vi "EditUser-Window.vi"(8 "error in":errorcluster, 9 "权  限":T1, 10 "密  码":string, 11 "用户名":string) -> (0 "error out":errorcluster)   [LabVIEW 2017, in "Login-UI.lvlib"]
uses:
  Login-UI.lvlib
  User-Role.ctl
  User-Info.ctl
panel:
  in  "Exit":bool
  in  "Save":bool
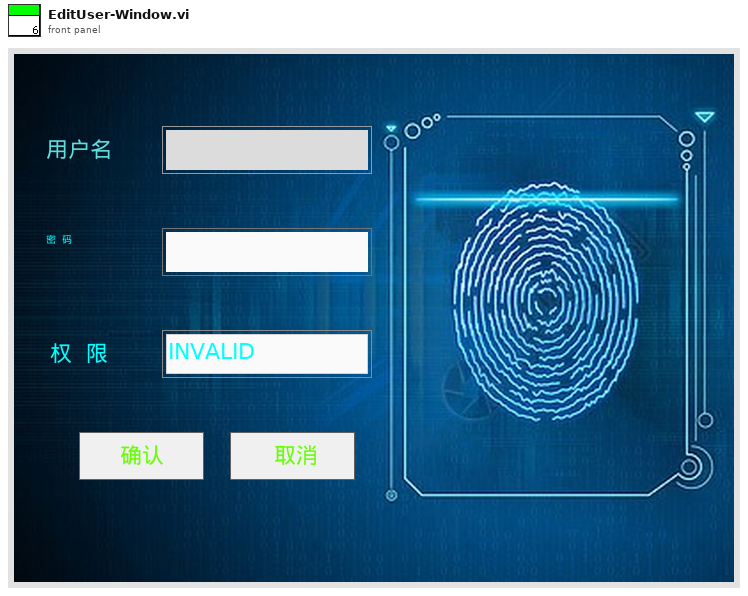
[diagram p1: front panel]
types:
  T1 = typedef "Login-UI.lvlib/User-Role.ctl" = enum16{"INVALID", "Operator", "Engineer", "Admin"}
  T2 = enum32{"Invalid", "Standard", "Closed", "Hidden", "Minimized", "Maximized"}
  T3 = enum32{"invalid app kind", "Development System", "Run Time System", "Student Edition", "Embedded LabVIEW", "Evaluation", "Custom"}
  T4 = typedef "Login-UI.lvlib/User-Info.ctl" = cluster{"UserName":string, "Password":string, "Role":T1}
  T5 = cluster{"Core":cluster{"Current VI Reference":refnum<vi>, "Close Panel on Exit?":bool}, "Your Boolean data":bool, "Your string data":string, "Cluster":T4}
  T6 = cluster{"Current VI Reference":refnum<vi>, "Close Panel on Exit?":bool}
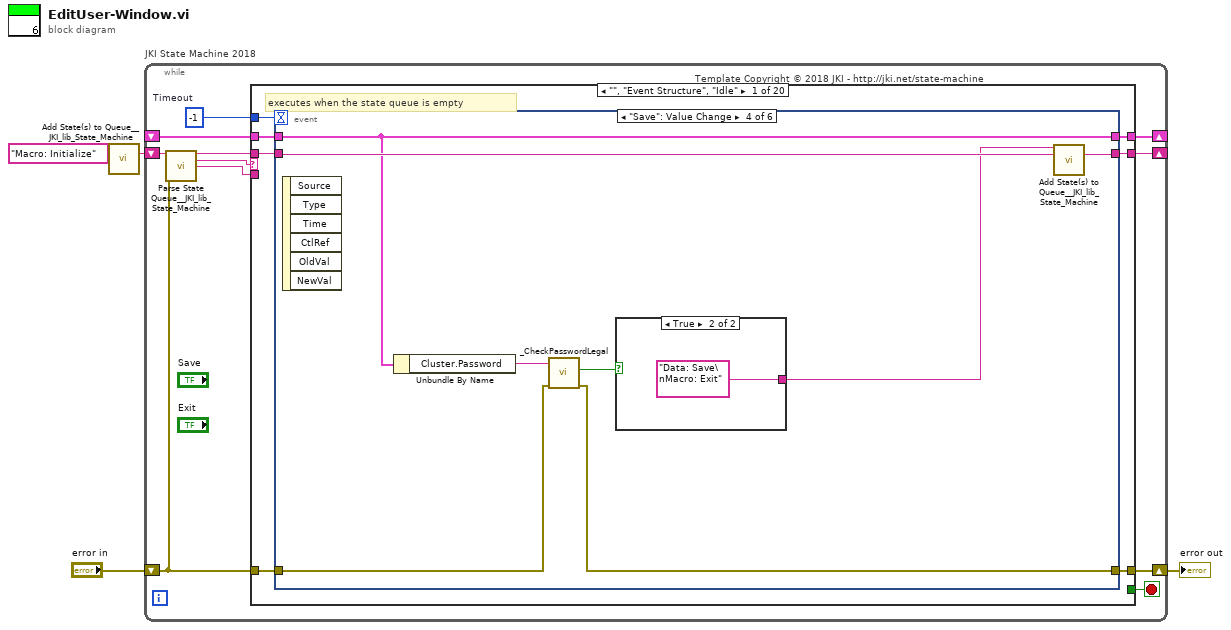
[diagram p0: block diagram]
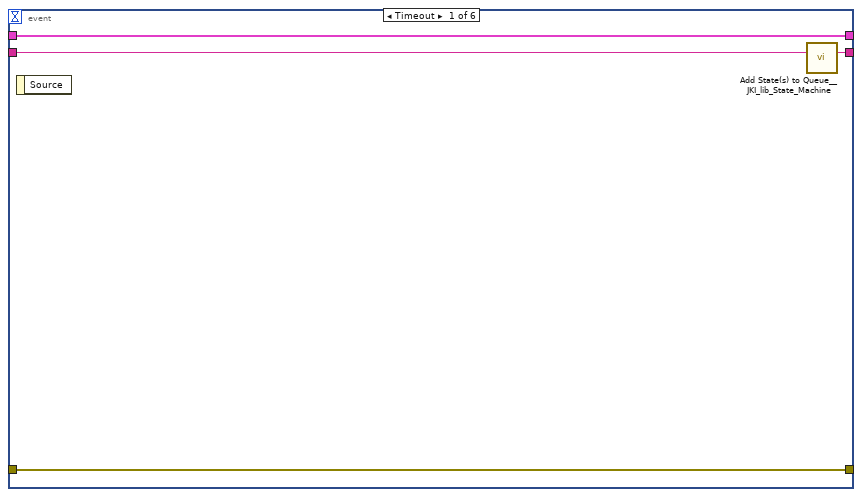
[diagram p2: hidden frame]
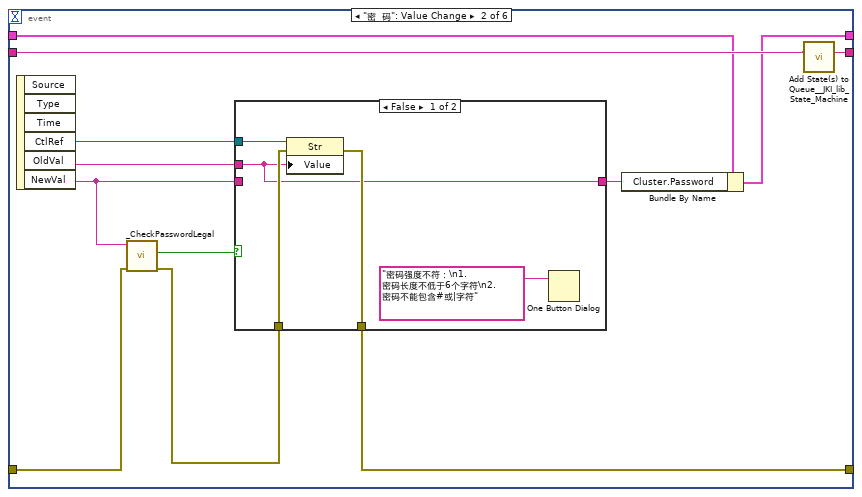
[diagram p3: hidden frame]
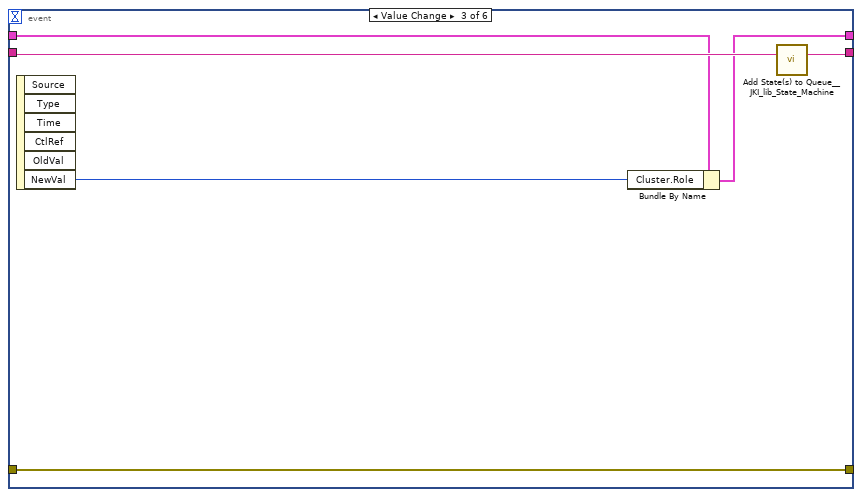
[diagram p5: hidden frame]
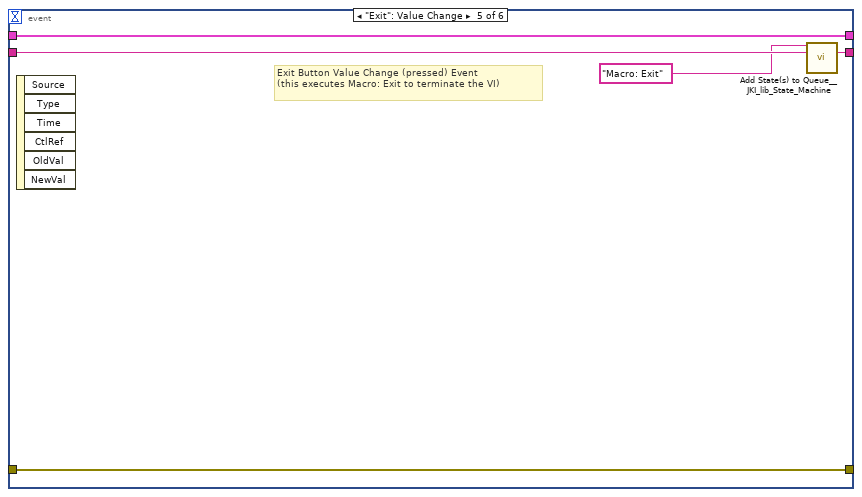
[diagram p7: hidden frame]
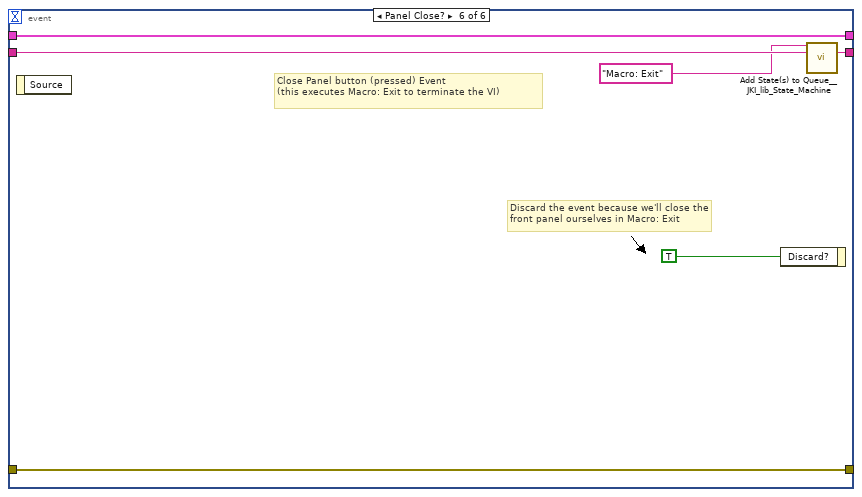
[diagram p8: hidden frame]
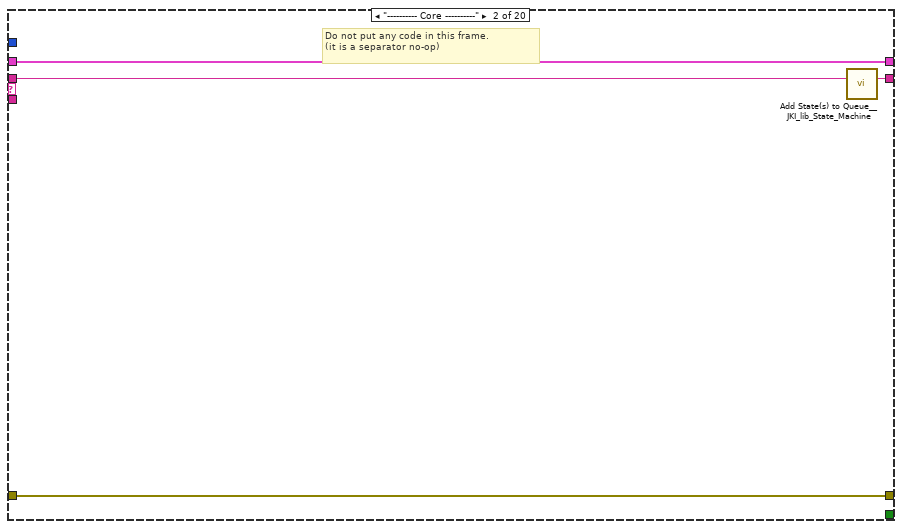
[diagram p9: hidden frame]
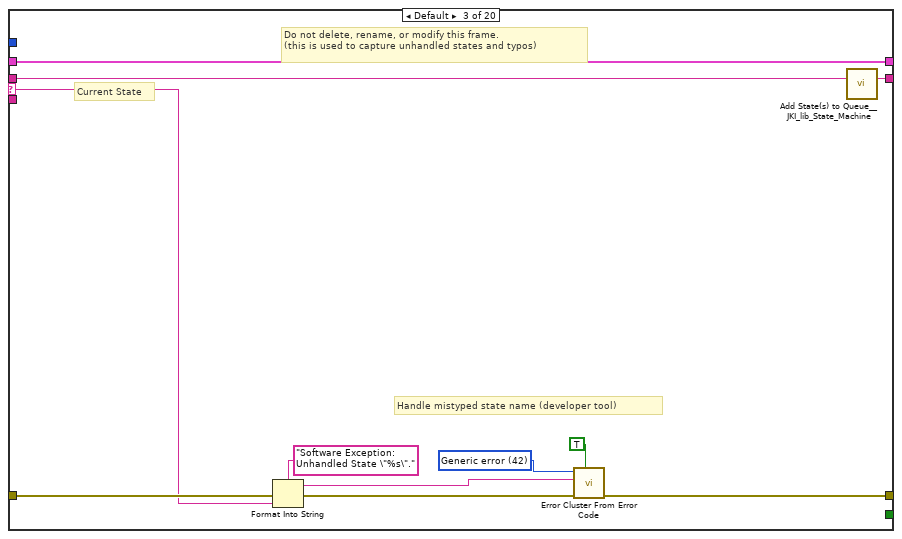
[diagram p10: hidden frame]
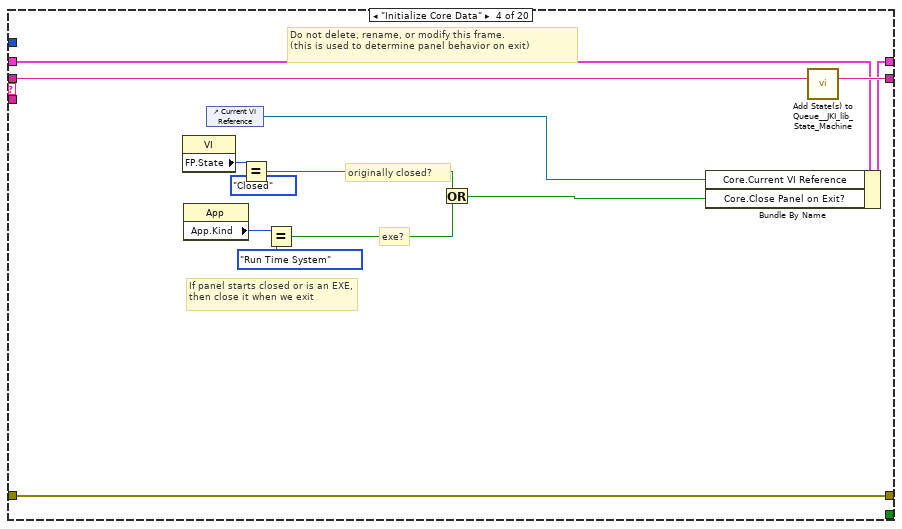
[diagram p11: hidden frame]
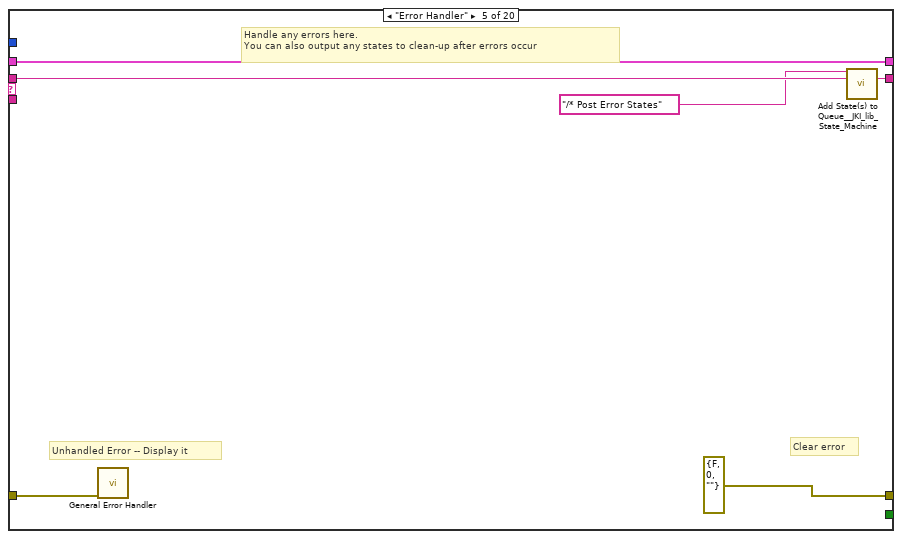
[diagram p12: hidden frame]
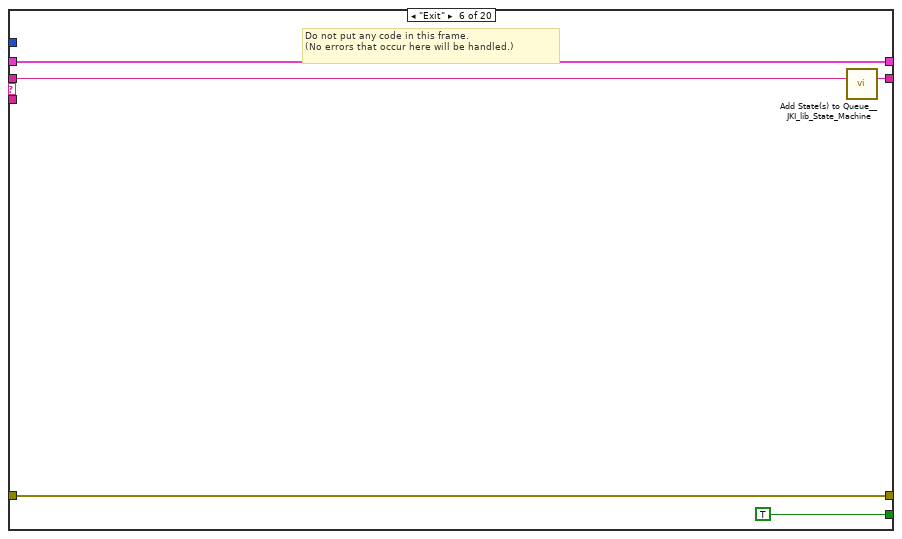
[diagram p13: hidden frame]
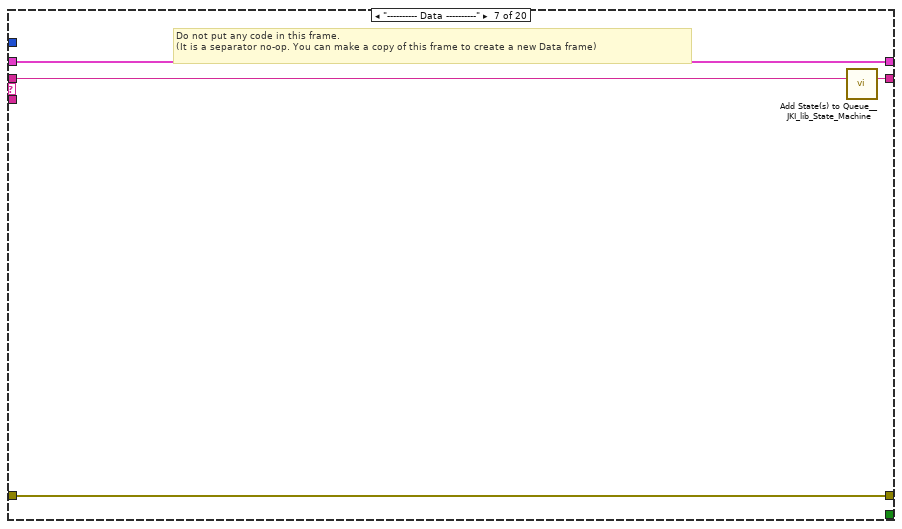
[diagram p14: hidden frame]
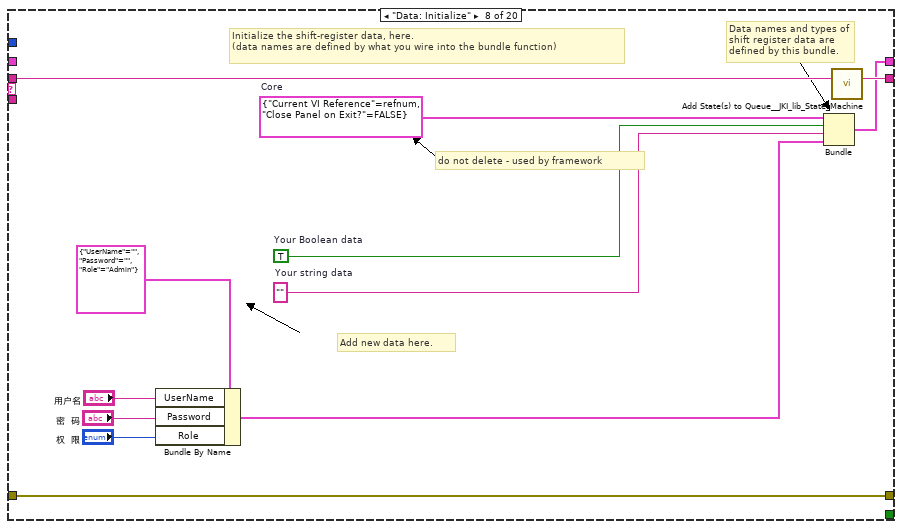
[diagram p15: hidden frame]
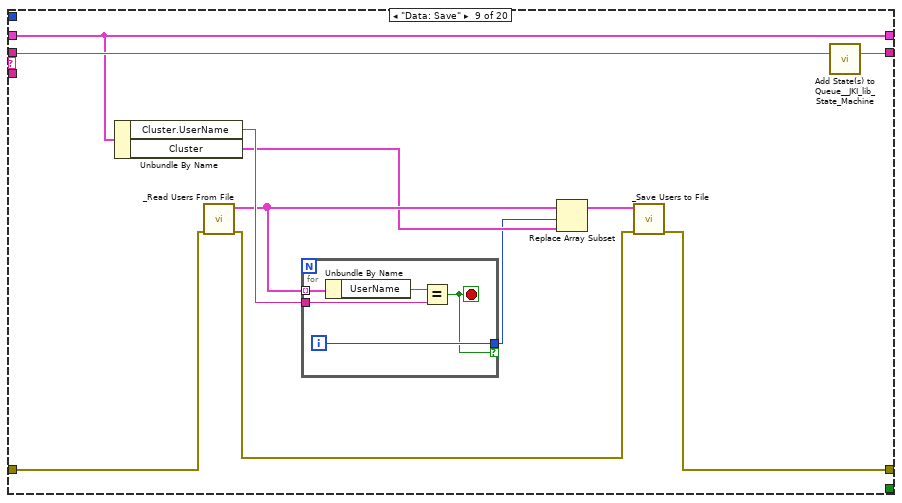
[diagram p16: hidden frame]
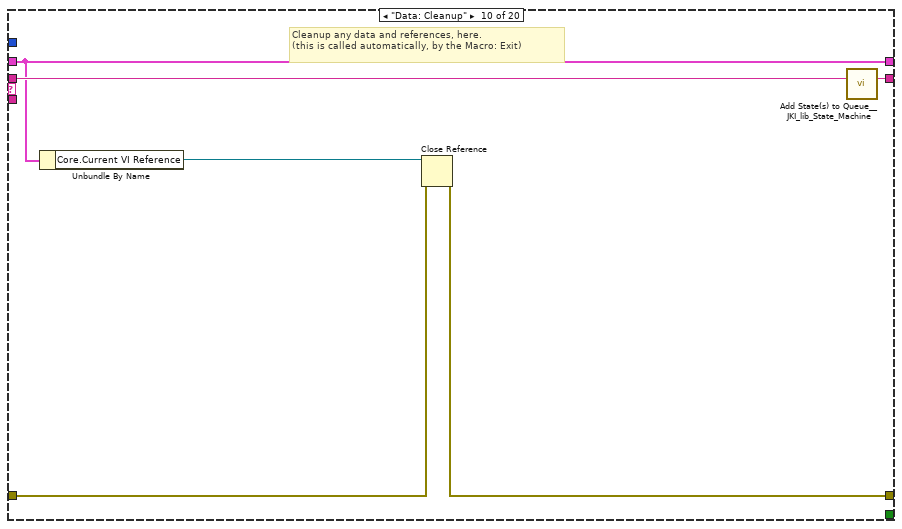
[diagram p17: hidden frame]
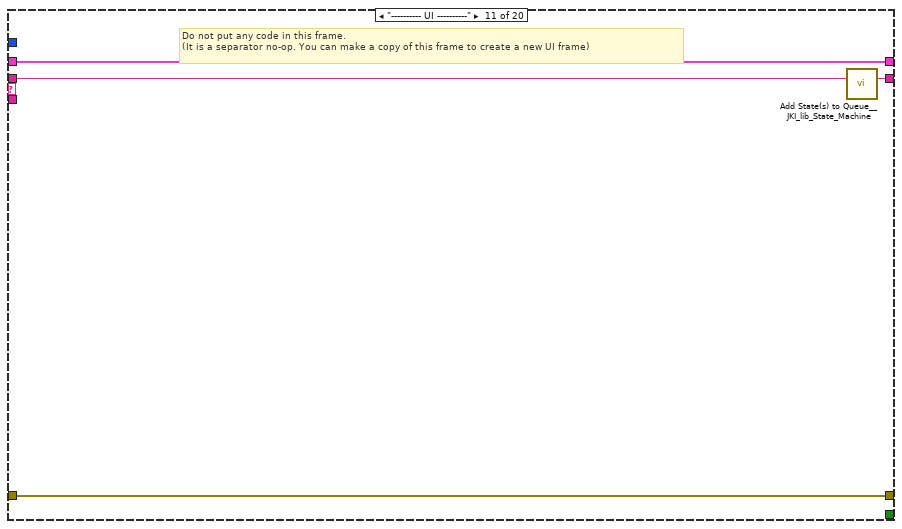
[diagram p18: hidden frame]
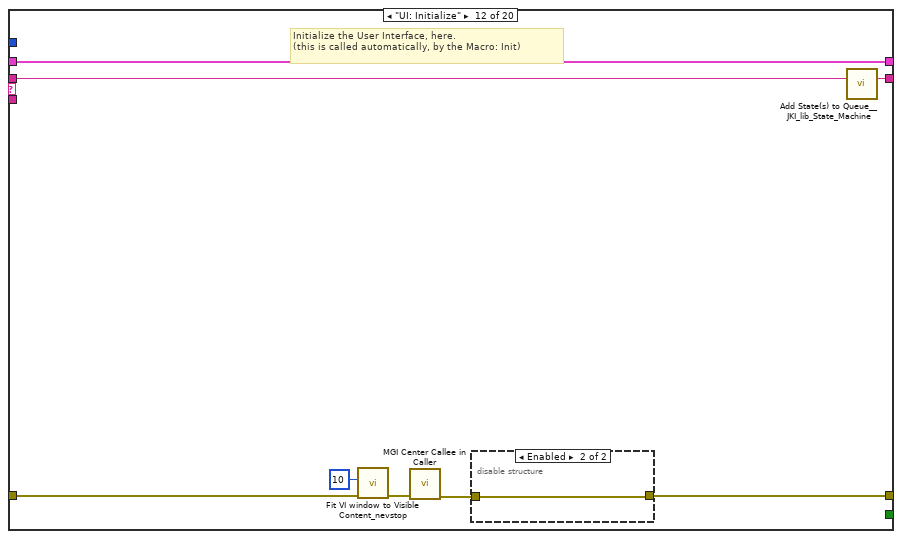
[diagram p19: hidden frame]
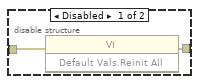
[diagram p20: hidden frame]
diagram:
  n1 = call <vilib>:"Add State(s) to Queue__JKI_lib_State_Machine.vi"("State(s) in (\"\")"="Macro: Initialize") -> ("States Out"=w4:string)  [unwired: 14 in]
  n2 = while "JKI State Machine 2018" {
    shift-right: [w8] -> _
    shift-left: _ -> [w7]
    shift-right: [w11] -> w1
    shift-left: "error in" -> [w5]
    shift-right: [w10] -> _
    shift-left: w4 -> [w12]
    stop <- w9 stop-if-true
    w6 = -1  # Timeout
    # "Template Copyright © 2018 JKI - http://jki.net/state-machine"
    n3 = call <vilib>:"Parse State Queue__JKI_lib_State_Machine.vi"("State Queue"=w12, "Error In (no error)"=w5) -> ("Remaining States"=w14:string, "Current State"=w15:string, "Arguments"=w13:string)  [unwired: 11 in]
    n4 = case shown="\"\", \"Event Structure\", \"Idle\"" w15 {
      selector: w15 -> [_ _ w76 _ _ _ _ _ _ _ _ _ _ _ _ _ _ _ _ _]
      tunnel: w14 -> [w22 w75 w80 w99 w105 w110 w114 w126 w136 w148 w152 w160 w169 w180 w249 w254 w264 w268 w272 w276]
      tunnel: w13 -> [_ _ _ _ _ _ _ _ _ _ _ _ w164 w174 _ _ _ _ _ _]
      tunnel: w7 -> [w21 w72 w78 w92 w102 w108 w111 _ w135 w143 w149 w158 w167 w176 w246 w251 w261 w265 w269 w273]
      tunnel: [w20 w73 w82 w96 errorcluster {"status"=FALSE, "code"=0, "source"=""} ("error out") w107 w112 w123 w133 w144 w150 w153 w165 w177 w247 w252 w262 w266 w270 w274] -> w11
      tunnel: w5 -> [w19 w73 w81 w96 w101 w107 w112 w123 w134 w145 w150 w155 w166 w178 w247 w252 w262 w266 w270 w274]
      tunnel: [w16 w74 w79 w98 w104 w109 w113 w125 w137 w147 w151 w159 w168 w179 w248 w253 w263 w267 w271 w275] -> w10
      tunnel: [_ _ _ _ _ TRUE _ _ _ _ _ _ _ _ _ _ _ _ _ _] -> w9
      tunnel: [w18 w72 w78 w97 w102 w108 w111 w124 w135 w143 w149 w158 w167 w176 w246 w251 w261 w265 w269 w273] -> w8
      tunnel: w6 -> [w17 _ _ _ _ _ _ _ _ _ _ _ _ _ _ _ _ _ _ _]
      frame "", "Event Structure", "Idle" {
        # "executes when the state queue is empty"
        n5 = event shown="[3] \"Save\": Value Change" {
          selector: _ -> [_ _ _ _ _ _]
          dyn-events: _ -> [_ _ _ _ _ _]
          timeout: w17 -> [_ _ _ _ _ _]
          tunnel: w22 -> [w26 w34 w49 w58 w65 w71]
          tunnel: [w25 w35 w50 w59 w64 w70] -> w16
          tunnel: w21 -> [w23 w29 w48 w56 w62 w68]
          tunnel: [w24 w36 w51 w52 w63 w69] -> w20
          tunnel: w19 -> [w24 w32 w51 w53 w63 w69]
          tunnel: [w23 w27 w47 w56 w62 w68] -> w18
          event Timeout {
            n6 = event-data() -> ()  [unwired: 1 in, 1 out]
            n7 = call <vilib>:"Add State(s) to Queue__JKI_lib_State_Machine.vi"("State(s) in (\"\")"=w26) -> ("States Out"=w25:string)  [unwired: 14 in]
          }
          event "密  码": Value Change {
            n8 = event-data() -> ("CtlRef"=w37:refnum<vi>, "OldVal"=w38:string, "NewVal"=w33:string)  [unwired: 1 in, 3 out]
            n9 = call "_CheckPasswordLegal.vi"("error in (no error)"=w32, "Password"=w33) -> ("error out"=w31:errorcluster, "legal?"=w30:bool)  [unwired: 8 in]
            n10 = case shown="False" w30 {
              tunnel: w38 -> [w39 _]
              tunnel: w33 -> [_ w44]
              tunnel: [w42 w45] -> w36
              tunnel: w37 -> [w41 _]
              tunnel: w31 -> [w40 w45]
              tunnel: [w39 w44] -> w28
              frame False {
                n11 = property class="Str"(reference=w41, error in=w40, "Value"=w39) -> (error out=w42:errorcluster)  [unwired: 1 out]
                n12 = One Button Dialog(message="密码强度不符：\n1.密码长度不低于6个字符\n2. 密码不能包含#或|字符") -> ()  [unwired: 1 in, 1 out]
              }
              frame True {
              }
            }
            n13 = Bundle By Name(cluster=w29, "Cluster.Password"=w28) -> (w27:T5)
            n14 = call <vilib>:"Add State(s) to Queue__JKI_lib_State_Machine.vi"("State(s) in (\"\")"=w34) -> ("States Out"=w35:string)  [unwired: 14 in]
          }
          event Value Change {
            n15 = event-data() -> ("NewVal"=w46:T1)  [unwired: 1 in, 5 out]
            n16 = Bundle By Name(cluster=w48, "Cluster.Role"=w46) -> (w47:T5)
            n17 = call <vilib>:"Add State(s) to Queue__JKI_lib_State_Machine.vi"("State(s) in (\"\")"=w49) -> ("States Out"=w50:string)  [unwired: 14 in]
          }
          event "Save": Value Change {
            n18 = event-data() -> ()  [unwired: 1 in, 6 out]
            n19 = Unbundle By Name(w56) -> ("Cluster.Password"=w57:string)
            n20 = call "_CheckPasswordLegal.vi"("error in (no error)"=w53, "Password"=w57) -> ("error out"=w52:errorcluster, "legal?"=w54:bool)  [unwired: 8 in]
            n21 = case shown="True" w54 {
              tunnel: [_ "Data: Save\nMacro: Exit"] -> w55
              frame False {
              }
              frame True {
              }
            }
            n22 = call <vilib>:"Add State(s) to Queue__JKI_lib_State_Machine.vi"("State(s) in Front (\"\")"=w55, "State(s) in (\"\")"=w58) -> ("States Out"=w59:string)  [unwired: 13 in]
          }
          event "Exit": Value Change {
            # "Exit Button Value Change (pressed) Event\n(this executes Macro: Exit to terminate the VI)"
            n23 = event-data() -> ()  [unwired: 1 in, 6 out]
            n24 = call <vilib>:"Add State(s) to Queue__JKI_lib_State_Machine.vi"("State(s) in Front (\"\")"="Macro: Exit", "State(s) in (\"\")"=w65) -> ("States Out"=w64:string)  [unwired: 13 in]
          }
          event Panel Close? {
            # "Discard the event because we'll close the front panel ourselves in Macro: Exit"
            # "Close Panel button (pressed) Event\n(this executes Macro: Exit to terminate the VI)"
            n25 = event-data() -> ()  [unwired: 1 in, 1 out]
            n26 = event-data("Discard?"=TRUE) -> ()  [unwired: 1 in, 1 out]
            n27 = call <vilib>:"Add State(s) to Queue__JKI_lib_State_Machine.vi"("State(s) in Front (\"\")"="Macro: Exit", "State(s) in (\"\")"=w71) -> ("States Out"=w70:string)  [unwired: 13 in]
          }
        }
      }
      frame "---------- Core ----------" {
        # "Do not put any code in this frame.\n(it is a separator no-op)"
        n28 = call <vilib>:"Add State(s) to Queue__JKI_lib_State_Machine.vi"("State(s) in (\"\")"=w75) -> ("States Out"=w74:string)  [unwired: 14 in]
      }
      frame Default {
        w85 = 42 items=["No error", "Argument error", "Memory is full", "Out of zone", "End of file", "File already open", "Generic file I/O error", "File not found", "File permission error", "Disk is full", "Duplicate path", "Too many files open", "System feature not enabled", "Resource file not found", "Cannot add resource", "Resource not found", "Image not found", "Image memory error", "Pen does not exist", "Config type invalid", "Config token not found", "Config parse error", "Config memory error", "Bad external code format", "Bad external code offset", "External code not present", "Null window", "Destroy window error", "Null menu", "Print aborted", "Bad print record", "Print driver error", "Windows error during printing", "Memory error during printing", "Print dialog error", "Generic print error", "Invalid device refnum", "Device not found", "Device parameter error", "Device unit error", "Cannot open device", "Device call aborted", "Generic error", "Cancelled by user", "Object ID too low", "Object ID too high", "Object not in heap", "Unknown heap", "Unknown object (invalid DefProc)", "Unknown object (DefProc not in table)", "Message out of range", "Invalid (null) method", "Unknown message", "Manager call not supported", "Bad address", "Network operation in progress", "Network operation timed out", "Connection is busy", "Network attribute not supported", "Network error", "Address in use", "System out of memory", "Connection aborted", "Connection refused", "Not connected", "Already connected", "Connection closed", "Initialization error (interapplication manager)", "Bad occurrence", "Wait on unbound occurrence handler", "Occurrence queue overflow", "Datalog type conflict", "Unused", "Unrecognized type (interapplication manager)", "Memory corrupt", "Failed to make temporary DLL", "Old CIN version", "Drag socket not found", "Failed to load drop-object", "Failed to register OLE object", "Failed to release OLE object", "Format specifier type mismatch", "Unknown format specifier", "Too few format specifiers", "Too many format specifiers", "Scan failed", "Newer CIN version", "Error converting to variant", "Runtime menu error", "Password tampered", "Variant attribute not found", "Incompatible variant data type", "Event data is not available", "Event Store is not present", "Occurrence is not found", "Event Queue is not created", "Event info is not available", "Refnum passed is NULL", "Error retrieving Class GUID", "Error retrieving CoClass GUID", "Error retrieving TypeLib GUID.", "Bad built application magic bytes.", "Specific driver is different from the specific driver associated with the Logical Name.", "There is no session opened to the class driver.", "Max Error", "MAX - Error with config objects", "MAX - Error loading configuration", "MAX - Group not supported"]
        # "Current State"
        # "Do not delete, rename, or modify this frame.\n(this is used to capture unhandled states and typos)"
        # "Handle mistyped state name (developer tool)"
        n29 = Format Into String(format string="Software Exception: Unhandled State \"%s\"." ("message"), error in=w81, w76) -> (resulting string=w84:string, error out=w83:errorcluster)  [unwired: 1 in]
        n30 = call <vilib>:"Error Cluster From Error Code.vi"("show call chain? (False)"=TRUE, "error in (no error)"=w83, "error message (\"\")"=w84, "error code (0)"=w85) -> ("error out"=w82:errorcluster)  [unwired: 5 in]
        n31 = call <vilib>:"Add State(s) to Queue__JKI_lib_State_Machine.vi"("State(s) in (\"\")"=w80) -> ("States Out"=w79:string)  [unwired: 14 in]
      }
      frame "Initialize Core Data" {
        # "Do not delete, rename, or modify this frame.\n(this is used to determine panel behavior on exit)"
        # "originally closed?"
        # "exe?"
        # "If panel starts closed or is an EXE, then close it when we exit"
        n32 = property class="VI"() -> ("FP.State"=w89:T2)  [unwired: 2 in, 2 out]
        n33 = property class="App"() -> ("App.Kind"=w95:T3)  [unwired: 2 in, 2 out]
        n34 = control-ref of="Current VI Reference"() -> (w90:refnum<vi>)
        n35 = Equal?(x=w89, y=T2."Closed" ("Front Panel Window:State")) -> (x = y?=w87:bool)
        n36 = Equal?(x=w95, y=T3."Run Time System" ("Application:Kind")) -> (x = y?=w93:bool)
        n37 = Or(x=w87, y=w93) -> (x .or. y?=w91:bool)
        n38 = Bundle By Name(cluster=w92, "Core.Current VI Reference"=w90, "Core.Close Panel on Exit?"=w91) -> (w97:T5)
        n39 = call <vilib>:"Add State(s) to Queue__JKI_lib_State_Machine.vi"("State(s) in (\"\")"=w99) -> ("States Out"=w98:string)  [unwired: 14 in]
      }
      frame "Error Handler" {
        # "Unhandled Error -- Display it"
        # "Handle any errors here.\nYou can also output any states to clean-up after errors occur"
        # "Clear error"
        n40 = call <vilib>:"General Error Handler.vi"("error in (no error)"=w101) -> ()  [unwired: 10 in, 5 out]
        n41 = call <vilib>:"Add State(s) to Queue__JKI_lib_State_Machine.vi"("State(s) in Front (\"\")"="/* Post Error States", "State(s) in (\"\")"=w105) -> ("States Out"=w104:string)  [unwired: 13 in]
      }
      frame "Exit" {
        # "Do not put any code in this frame.\n(No errors that occur here will be handled.)"
        n42 = call <vilib>:"Add State(s) to Queue__JKI_lib_State_Machine.vi"("State(s) in (\"\")"=w110) -> ("States Out"=w109:string)  [unwired: 14 in]
      }
      frame "---------- Data ----------" {
        # "Do not put any code in this frame.\n(It is a separator no-op. You can make a copy of this frame to create a new Data frame)"
        n43 = call <vilib>:"Add State(s) to Queue__JKI_lib_State_Machine.vi"("State(s) in (\"\")"=w114) -> ("States Out"=w113:string)  [unwired: 14 in]
      }
      frame "Data: Initialize" {
        w120 = T6 {"Current VI Reference"=refnum, "Close Panel on Exit?"=FALSE}  # Core
        w122 = TRUE  # Your Boolean data
        w121 = ""  # Your string data
        # "do not delete - used by framework"
        # "Add new data here."
        # "Data names and types of shift register data are defined by this bundle."
        # "Initialize the shift-register data, here.\n(data names are defined by what you wire into the bundle function)"
        n44 = Bundle By Name(cluster=T4 {"UserName"="", "Password"="", "Role"=enum."Admin"} ("Cluster"), "UserName"="用户名", "Password"="密  码", "Role"="权  限") -> (w115:T4)
        n45 = Bundle("Core"=w120, "Your Boolean data"=w122, "Your string data"=w121, "Cluster"=w115) -> (w124:T5)  [unwired: 1 in]
        n46 = call <vilib>:"Add State(s) to Queue__JKI_lib_State_Machine.vi"("State(s) in (\"\")"=w126) -> ("States Out"=w125:string)  [unwired: 14 in]
      }
      frame "Data: Save" {
        n47 = Unbundle By Name(w135) -> ("Cluster.UserName"=w131:string, "Cluster"=w129:T4)
        n48 = call "_Read Users From File.vi"("Error in"=w134) -> ("Error out"=w132:errorcluster, "Array"=w130:T4[])  [unwired: 9 in]
        n49 = for {
          tunnel: w130 -> [w142] mode=indexing
          tunnel: w131 -> [w140]
          tunnel: [w139] -> w128 if=w138
          i -> [w139]
          stop <- w138 stop-if-true
          n50 = Unbundle By Name(w142) -> ("UserName"=w141:string)
          n51 = Equal?(x=w141, y=w140) -> (x = y?=w138:bool)
        }
        n52 = Replace Array Subset(array=w130, new element=w129, index=w128) -> (w127:T4[])
        n53 = call "_Save Users to File.vi"("Error in"=w132, "Array"=w127) -> ("Error out"=w133:errorcluster)  [unwired: 9 in]
        n54 = call <vilib>:"Add State(s) to Queue__JKI_lib_State_Machine.vi"("State(s) in (\"\")"=w136) -> ("States Out"=w137:string)  [unwired: 14 in]
      }
      frame "Data: Cleanup" {
        # "Cleanup any data and references, here.\n(this is called automatically, by the Macro: Exit)"
        n55 = Unbundle By Name(w143) -> ("Core.Current VI Reference"=w146:refnum<vi>)
        n56 = Close Reference(reference=w146, error in (no error)=w145) -> (error out=w144:errorcluster)
        n57 = call <vilib>:"Add State(s) to Queue__JKI_lib_State_Machine.vi"("State(s) in (\"\")"=w148) -> ("States Out"=w147:string)  [unwired: 14 in]
      }
      frame "---------- UI ----------" {
        # "Do not put any code in this frame.\n(It is a separator no-op. You can make a copy of this frame to create a new UI frame)"
        n58 = call <vilib>:"Add State(s) to Queue__JKI_lib_State_Machine.vi"("State(s) in (\"\")"=w152) -> ("States Out"=w151:string)  [unwired: 14 in]
      }
      frame "UI: Initialize" {
        # "Initialize the User Interface, here.\n(this is called automatically, by the Macro: Init)"
        n59 = call <userlib>:"Fit VI window to Visible Content_nevstop.vi"("error in (no error)"=w155, "border spacing (2 px)"=10) -> ("error out"=w157:errorcluster)  [unwired: 4 in, 1 out]
        n60 = call <userlib>:"MGI Center Callee in Caller.vi"("Error In"=w157) -> ("Error Out"=w154:errorcluster)  [unwired: 10 in]
        n61 = disable-structure shown="Enabled" {
          disable-tunnel: w154 -> [w162 w163]
          disable-tunnel: [w161 w163] -> w153
          frame Disabled {
            n62 = invoke class="VI" method="Default Vals.Reinit All"(error in=w162) -> (error out=w161:errorcluster)  [unwired: 2 in, 2 out]
          }
          frame Enabled {
          }
        }
        n63 = call <vilib>:"Add State(s) to Queue__JKI_lib_State_Machine.vi"("State(s) in (\"\")"=w160) -> ("States Out"=w159:string)  [unwired: 14 in]
      }
      frame "UI: Cursor Set" {
        # "Argument"
        # "Set and Unset Cursor Busy.\n(Usage: \"UI: Cursor Set >> Busy|Idle\")"
        n64 = case shown="\"Idle\", Default" w164 {
          tunnel: w166 -> [w171 w173]
          tunnel: [w170 w172] -> w165
          frame "Idle", Default {
            n65 = call <vilib>:"Unset Busy.vi"("error in (no error)"=w171) -> ("error out"=w170:errorcluster)  [unwired: 10 in]
          }
          frame "Busy" {
            n66 = call <vilib>:"Set Busy.vi"("error in (no error)"=w173) -> ("error out"=w172:errorcluster)  [unwired: 9 in, 1 out]
          }
        }
        n67 = call <vilib>:"Add State(s) to Queue__JKI_lib_State_Machine.vi"("State(s) in (\"\")"=w169) -> ("States Out"=w168:string)  [unwired: 14 in]
      }
      frame "UI: Front Panel State" {
        # "Argument"
        # "Set Front Panel Open or Closed\n(Usage: \"UI: Front Panel State >> Open|Close\")"
        n68 = Unbundle By Name(w176) -> ("Core.Current VI Reference"=w175:refnum<vi>)
        n69 = case shown="\"Minimize\", \"Minimized\"" w174 {
          tunnel: w178 -> [w186 w201 w212 w225 w238]
          tunnel: [w188 w202 w214 w227 w240] -> w177
          tunnel: w175 -> [w187 w199 w213 w226 w239]
          frame "Open", "Standard", Default {
            w181 = T2."Standard" ("State")
            n70 = property class="VI"(reference=w187, error in=w186) -> (reference out=w184:refnum<vi>, error out=w185:errorcluster, "FP.State"=w183:T2)
            n71 = Not Equal?(x=w183, y=w181) -> (x != y?=w182:bool)
            n72 = case shown="True" w182 {
              tunnel: [w192 w194] -> w188
              tunnel: w185 -> [w191 w194]
              tunnel: w184 -> [w190 _]
              tunnel: w181 -> [w189 _]
              frame True {
                n73 = invoke class="VI" method="FP.Open"(reference=w190, error in=w191, "Activate"=TRUE, "State"=w189) -> (error out=w192:errorcluster)  [unwired: 1 in, 4 out]
              }
              frame False {
              }
            }
          }
          frame "Close", "Closed" {
            n74 = property class="VI"(reference=w199, error in=w201) -> (reference out=w198:refnum<vi>, error out=w200:errorcluster, "FP.State"=w196:T2)
            n75 = Not Equal?(x=w196, y=T2."Closed" ("Front Panel Window:State")) -> (x != y?=w195:bool)
            n76 = case shown="True" w195 {
              tunnel: [w203 w206] -> w202
              tunnel: w200 -> [w203 w205]
              tunnel: w198 -> [_ w204]
              frame False {
              }
              frame True {
                n77 = invoke class="VI" method="FP.Close"(reference=w204, error in=w205) -> (error out=w206:errorcluster)  [unwired: 1 in, 2 out]
              }
            }
          }
          frame "Hidden", "Hide" {
            w207 = T2."Hidden" ("State")
            n78 = property class="VI"(reference=w213, error in=w212) -> (reference out=w210:refnum<vi>, error out=w211:errorcluster, "FP.State"=w209:T2)
            n79 = Not Equal?(x=w209, y=w207) -> (x != y?=w208:bool)
            n80 = case shown="True" w208 {
              tunnel: [w218 w219] -> w214
              tunnel: w211 -> [w217 w219]
              tunnel: w210 -> [w216 _]
              tunnel: w207 -> [w215 _]
              frame True {
                n81 = invoke class="VI" method="FP.Open"(reference=w216, error in=w217, "State"=w215) -> (error out=w218:errorcluster)  [unwired: 2 in, 4 out]
              }
              frame False {
              }
            }
          }
          frame "Minimize", "Minimized" {
            w220 = T2."Minimized" ("State")
            n82 = property class="VI"(reference=w226, error in=w225) -> (reference out=w223:refnum<vi>, error out=w224:errorcluster, "FP.State"=w222:T2)
            n83 = Not Equal?(x=w222, y=w220) -> (x != y?=w221:bool)
            n84 = case shown="True" w221 {
              tunnel: [w231 w232] -> w227
              tunnel: w224 -> [w230 w232]
              tunnel: w223 -> [w229 _]
              tunnel: w220 -> [w228 _]
              frame True {
                n85 = invoke class="VI" method="FP.Open"(reference=w229, error in=w230, "State"=w228) -> (error out=w231:errorcluster)  [unwired: 2 in, 4 out]
              }
              frame False {
              }
            }
          }
          frame "Maximize", "Maximized" {
            w233 = T2."Maximized" ("State")
            n86 = property class="VI"(reference=w239, error in=w238) -> (reference out=w236:refnum<vi>, error out=w237:errorcluster, "FP.State"=w235:T2)
            n87 = Not Equal?(x=w235, y=w233) -> (x != y?=w234:bool)
            n88 = case shown="True" w234 {
              tunnel: [w244 w245] -> w240
              tunnel: w237 -> [w243 w245]
              tunnel: w236 -> [w242 _]
              tunnel: w233 -> [w241 _]
              frame True {
                n89 = invoke class="VI" method="FP.Open"(reference=w242, error in=w243, "State"=w241) -> (error out=w244:errorcluster)  [unwired: 2 in, 4 out]
              }
              frame False {
              }
            }
          }
        }
        n90 = call <vilib>:"Add State(s) to Queue__JKI_lib_State_Machine.vi"("State(s) in (\"\")"=w180) -> ("States Out"=w179:string)  [unwired: 14 in]
      }
      frame "---------- Macro ----------" {
        # "Do not put any code in this frame.\n(It is a separator no-op. You can make a copy of this frame to create a new Macro frame)"
        n91 = call <vilib>:"Add State(s) to Queue__JKI_lib_State_Machine.vi"("State(s) in (\"\")"=w249) -> ("States Out"=w248:string)  [unwired: 14 in]
      }
      frame "Macro: Initialize" {
        w250 = "Data: Initialize\nInitialize Core Data\nUI: Initialize\nUI: Front Panel State >> Open"  # Data: Initialize Initialize Core Data UI: Initialize UI: Front Panel State >> Open
        # "Initialization Macro\n(This is called once, when the VI starts)"
        n92 = call <vilib>:"Add State(s) to Queue__JKI_lib_State_Machine.vi"("State(s) in Front (\"\")"=w250, "State(s) in (\"\")"=w254) -> ("States Out"=w253:string)  [unwired: 13 in]
      }
      frame "Macro: Exit" {
        # "Exit Macro\n(This is called once, when the VI exits)"
        n93 = Unbundle By Name(w261) -> ("Core.Close Panel on Exit?"=w260:bool)
        n94 = Select(t="UI: Front Panel State >> Close", s=w260, f="") -> (s? t:f=w257:string)
        n95 = call <vilib>:"Add State(s) to Queue__JKI_lib_State_Machine.vi"("State(s) in (\"\")"=w257, "State(s) at Back (\"\")"="Data: Cleanup\nExit") -> ("States Out"=w255:string)  [unwired: 13 in]
        n96 = call <vilib>:"Add State(s) to Queue__JKI_lib_State_Machine.vi"("State(s) in Front (\"\")"=w255, "State(s) in (\"\")"=w264) -> ("States Out"=w263:string)  [unwired: 13 in]
      }
      frame "---------- New Category ----------" {
        # "Template Separator\n(You can make a copy of, or modify, this frame)"
        n97 = call <vilib>:"Add State(s) to Queue__JKI_lib_State_Machine.vi"("State(s) in (\"\")"=w268) -> ("States Out"=w267:string)  [unwired: 14 in]
      }
      frame "New Category: 1" {
        # "Your code here.\n(You can make a copy of, or modify, this frame)"
        n98 = call <vilib>:"Add State(s) to Queue__JKI_lib_State_Machine.vi"("State(s) in (\"\")"=w272) -> ("States Out"=w271:string)  [unwired: 14 in]
      }
      frame "New Category: 2" {
        # "Your code here.\n(You can make a copy of, or modify, this frame)"
        n99 = call <vilib>:"Add State(s) to Queue__JKI_lib_State_Machine.vi"("State(s) in (\"\")"=w276) -> ("States Out"=w275:string)  [unwired: 14 in]
      }
    }
  }
  "error out" <- w1
